vi "Calculate start and stop.vi"(8 "error in (no error)":errorcluster, 11 "Autofocus in":refnum<class "Autofocus.lvclass">) -> (0 "error out":errorcluster, 3 "Autofocus out":refnum<class "Autofocus.lvclass">)   [LabVIEW 2012, in "Autofocus.lvclass"]
uses:
  Autofocus.lvclass
  Autofocus.lvclass/Autofocus.ctl
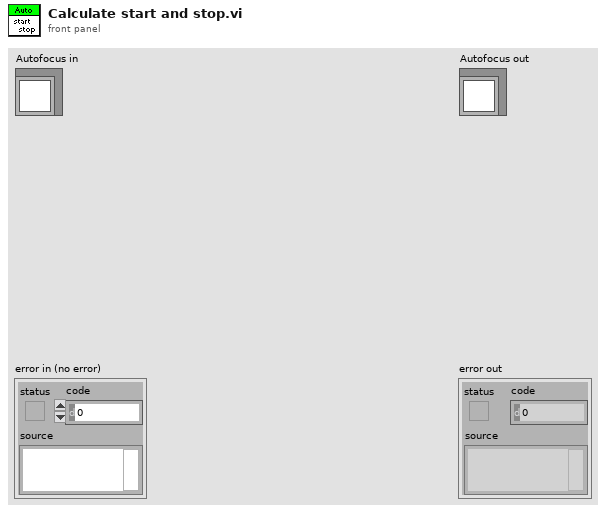
[diagram p1: front panel]
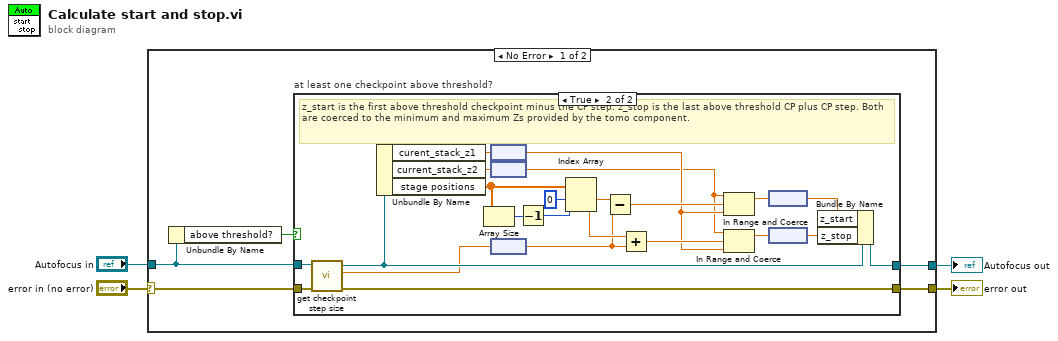
[diagram p0: block diagram]
diagram:
  n1 = case shown="No Error" "error in (no error)" {
    selector: "error in (no error)" -> [w8 w36]
    tunnel: [w7 w36] -> w3
    tunnel: [w9 w35] -> w1
    tunnel: "Autofocus in" -> [w6 w35]
    frame No Error {
      n2 = Unbundle By Name(w6) -> ("above threshold?"=w5:bool)
      n3 = case "at least one checkpoint above threshold?" shown="True" w5 {
        tunnel: [w11 w30] -> w9
        tunnel: w6 -> [w11 w29]
        tunnel: w8 -> [w10 w27]
        tunnel: [w10 w26] -> w7
        frame False {
        }
        frame True {
          # "z_start is the first above threshold checkpoint minus the CP step. z_stop is the last above threshold CP plus CP step. Both are coerced to the minimum and maximum Zs provided by the tomo component."
          n4 = call-dynamic "get checkpoint step size.vi"("error in (no error)"=w27, "Autofocus in"=w29) -> ("error out"=w26:errorcluster, "checkpoint stepsize"=w25:dbl[unit], "Autofocus out"=w28:refnum<class "Autofocus.lvclass">)  [unwired: 7 in]
          n5 = Unbundle By Name(w28) -> ("curent_stack_z1"=w15:dbl[unit], "current_stack_z2"=w13:dbl[unit], "stage positions"=w33:dbl[])
          n6 = Array Size(array=w33) -> (size(s)=w34:i32)
          n7 = node(w15) -> (w14:dbl)
          n8 = node(w13) -> (w12:dbl)
          n9 = node(w25) -> (w22:dbl)
          n10 = Decrement(x=w34) -> (x-1=w32:i32)
          n11 = Index Array(array=w33, index #1=0 ("index"), index #2=w32) -> (element #1=w23:dbl, element #2=w24:dbl)
          n12 = Subtract(x=w23, y=w22) -> (x-y=w20:dbl)
          n13 = Add(x=w24, y=w22) -> (x+y=w21:dbl)
          n14 = In Range and Coerce(upper limit=w12, x=w20, lower limit=w14) -> (coerced(x)=w17:dbl)  [unwired: 1 out]
          n15 = In Range and Coerce(upper limit=w12, x=w21, lower limit=w14) -> (coerced(x)=w19:dbl)  [unwired: 1 out]
          n16 = node(w17) -> (w16:dbl[unit])
          n17 = node(w19) -> (w18:dbl[unit])
          n18 = Bundle By Name(cluster=w28, "z_start"=w16, "z_stop"=w18) -> (w30:refnum<class "Autofocus.lvclass">)
        }
      }
    }
    frame Error {
    }
  }
  "error out" <- w3
  "Autofocus out" <- w1
